vi "SQLite Connection Probe.vi"(11 "Connection in":refnum<class "Connection.lvclass">) -> (2 "Value String":string, 3 "Boolean":bool)   [LabVIEW 2023, in "SQLite.lvlib" / "Connection.lvclass"]
uses:
  Connection.lvclass
panel:
  out "text":string
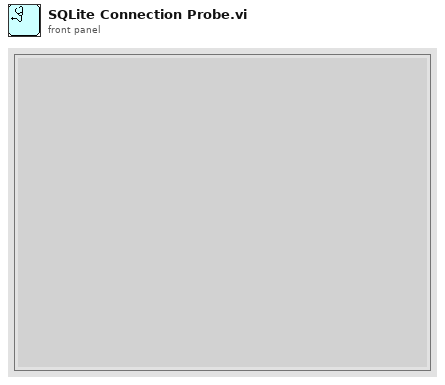
[diagram p1: front panel]
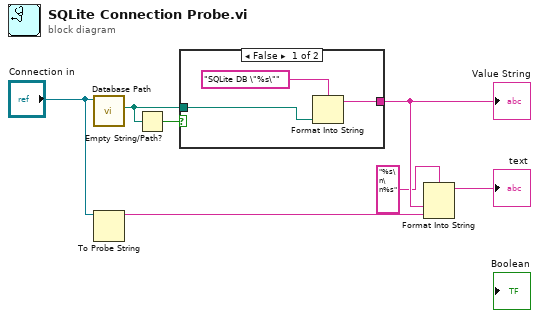
[diagram p0: block diagram]
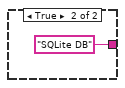
[diagram p2: hidden frame]
diagram:
  n1 = call "Database Path.vi"("Connection in"="Connection in") -> ("Path to Database"=w5:path)  [unwired: 8 in, 2 out]
  n2 = To Probe String(7:"Connection in") -> (3:w2:string)  [unwired: 2 in, 1 out]
  n3 = Empty String/Path?(string/path=w5) -> (empty?=w6:bool)
  n4 = case shown="False" w6 {
    tunnel: [w9 "SQLite DB"] -> w4
    tunnel: w5 -> [w8 _]
    frame False {
      n5 = Format Into String(format string="SQLite DB \"%s\"", w8) -> (resulting string=w9:string)  [unwired: 2 in, 1 out]
    }
    frame True {
    }
  }
  "Value String" <- w4
  n6 = Format Into String(format string="%s\n\n%s", w4, w2) -> (resulting string=→"text":string)  [unwired: 2 in, 1 out]
